vi "rs3_ReadDepthPreference4.vi"(0 "file (use dialog)":path) -> (1 "HDAD 2*":T2={"lambdaCensus"=126.0, "lambdaAD"=800.0, "ignoreSAD"=0}, 2 "ST_AE_Control":cluster{"meanIntensitySetpoint":u32}={"meanIntensitySetpoint"=800}, 3 "ST Color Control 2":T5, 4 "depth control 2":T9={"plusIncrement (47)"=19, "MinusDecrement (46)"=4, "deepSeaMedianThreshold (48)"=554, "scoreThreshA(49)"=1, "scoreThreshB (50)"=632, "textureDifferenceThreshold (52)"=0, "textureCountThreshold (51)"=32, "deepSea2ndPeakThresh.(53)"=665, "deepSeaNeighborThresh.(54)"=126, "IrAgreeThreshold (55)"=11}, 6 "ST RSM 2":T8={"rsmBypass (56)"=0, "diffThresh (57)"=6.49, "sloRauDiffThresh(58)"=0.305, "removeThresh(59)"=60}, 8 "Depth Table":T1={"depthUnits, um"=1000, "depthClampMin"=0, "depthClampMax"=65535, "disparityMultiplier"=0, "disparityShift(0-127)"=0}, 9 "text":string="{\n    \"param-disableraucolor\": 0,\n    \"param-disablesadcolor\": 0,\n    \"param-disablesadnormalize\": 0,\n    \"param-disablesloleftcolor\": 0,\n    \"param-disableslorightcolor\": 0,\n    \"param-lambdaad\": 833,\n    \"param-lambdacensus\": 26,\n    \"param-leftrightthreshold\": 11,\n    \"param-maxscorethreshb\": 632,\n    \"param-medianthreshold\": 554,\n    \"param-minscorethresha\": 1,\n    \"param-neighborthresh\": 126,\n    \"param-raumine\": 7,\n    \"param-rauminn\": 1,\n    \"param-rauminnssum\": 7,\n    \"param-raumins\": 3,\n    \"param-rauminw\": 5,\n    \"param-rauminwesum\": 12,\n    \"param-regioncolorthresholdb\": 0.26379450841061053,\n    \"param-regioncolorthresholdg\": 0.9806201235330119,\n    \"param-regioncolorthresholdr\": 0.013826660558426103,\n    \"param-regionshrinku\": 4,\n    \"param-regionshrinkv\": 1,\n    \"param-regionspatialthresholdu\": 7,\n    \"param-regionspatialthresholdv\": 3,\n    \"param-robbinsmonrodecrement\": 4,\n    \"param-robbinsmonroincrement\": 19,\n    \"param-rsmdiffthreshold\": 1.0367311077984247,\n    \"param-rsmrauslodiffthreshold\": 0.8955340364089305,\n    \"param-rsmremovethreshold\": 0.7604262237190709,\n    \"param-scanlineedgetaub\": 105,\n    \"param-scanlineedgetaug\": 442,\n    \"param-scanlineedgetaur\": 46,\n    \"param-scanlinep1\": 93,\n    \"param-scanlinep1onediscon\": 70,\n    \"param-scanlinep1twodiscon\": 92,\n    \"param-scanlinep2\": 473,\n    \"param-scanlinep2onediscon\": 123,\n    \"param-scanlinep2twodiscon\": 409,\n    \"param-secondpeakdelta\": 665,\n    \"param-texturecountthresh\": 32,\n    \"param-texturedifferencethresh\": 0,\n    \"param-usersm\": 1\n}", 10 "ST SLO Penalty 2":T7={"sloK1Penalty (79)"=10, "sloK2Penalty (80)"=60, "sloK1PenaltyMod1(81)"=84, "sloK2PenaltyMod1(82)"=56, "sloK1PenaltyMod2(83)"=59, "sloK2PenaltyMod2(84)"=4}, 11 "ST_CensusEnable":cluster{"uDiameter":u32, "vDiameter":u32}={"uDiameter"=9, "vDiameter"=9}, 12 "ST SLO Threshold 2":T3={"SLOdiffThreshRed(76)"=200, "SLODiffThreshGreen(77)"=200, "SLODiffThreshBlue(78)"=200}, 13 "error out":errorcluster, 14 "ST Rau Threshold 2":T4={"rauDiffThreshRed(73)"=70, "rauDiffThreshGreen(74)"=70, "rauDiffThreshBlue(75)"=70}, 15 "ST RAU vector 2":T6={"minWest (60)"=7, "minEast (61)"=7, "minWEsum (62)"=12, "minNorth (63)"=3, "minSouth (64)"=2, "minNSSum(65)"=1, "uStrink (66)"=2, "vShrink (67)"=1})   [LabVIEW 2017, in "libRealSense3.lvlib"]
uses:
  libRealSense3.lvlib
panel:
  in  "error in (no error)":errorcluster
  # "RS2 Read Depth Preferences 4"
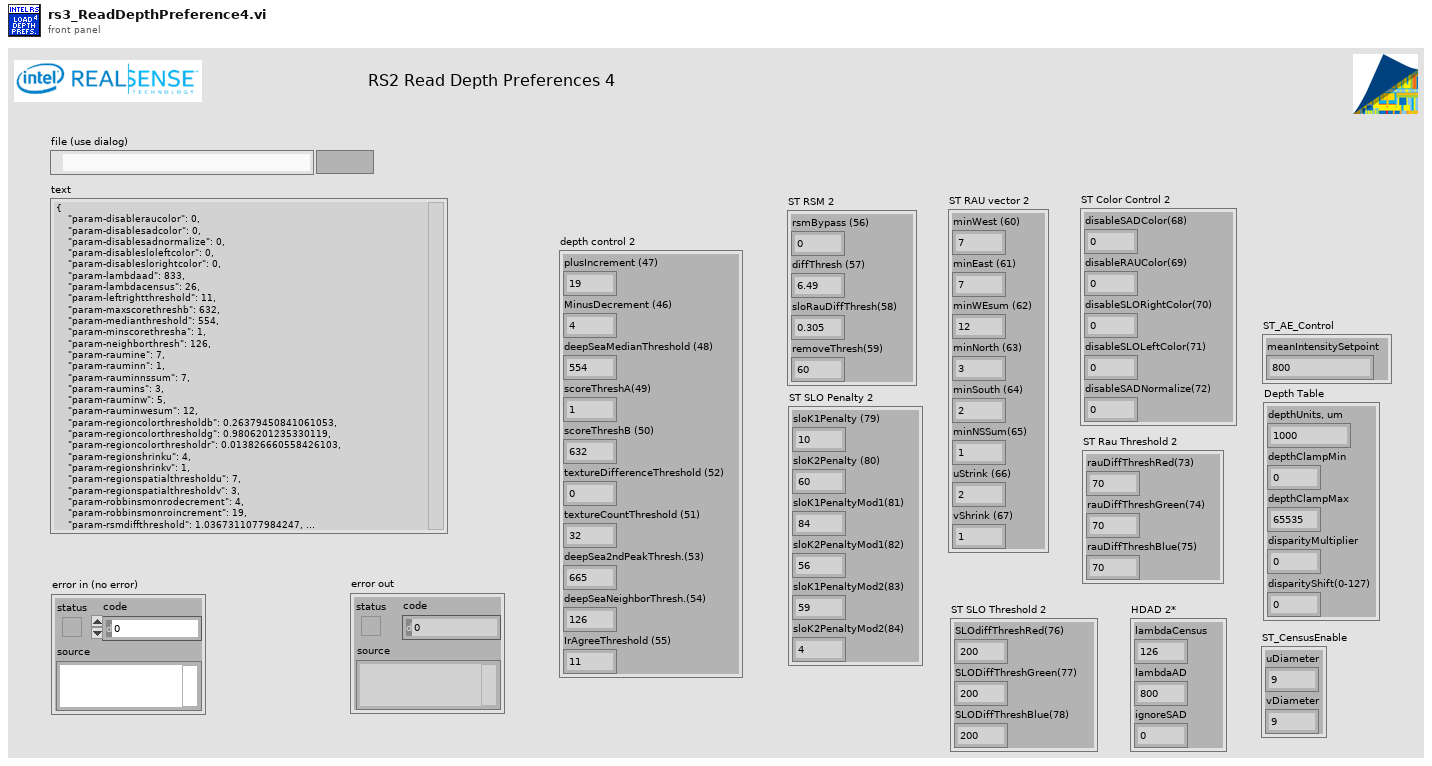
[diagram p1: front panel]
types:
  T1 = cluster{"depthUnits, um":u32, "depthClampMin":u32, "depthClampMax":u32, "disparityMultiplier":u32, "disparityShift(0-127)":u32}
  T2 = cluster{"lambdaCensus":sgl, "lambdaAD":sgl, "ignoreSAD":u32}
  T3 = cluster{"SLOdiffThreshRed(76)":u32, "SLODiffThreshGreen(77)":u32, "SLODiffThreshBlue(78)":u32}
  T4 = cluster{"rauDiffThreshRed(73)":u32, "rauDiffThreshGreen(74)":u32, "rauDiffThreshBlue(75)":u32}
  T5 = cluster{"disableSADColor(68)":u32, "disableRAUColor(69)":u32, "disableSLORightColor(70)":u32, "disableSLOLeftColor(71)":u32, "disableSADNormalize(72)":u32}
  T6 = cluster{"minWest (60)":u32, "minEast (61)":u32, "minWEsum (62)":u32, "minNorth (63)":u32, "minSouth (64)":u32, "minNSSum(65)":u32, "uStrink (66)":u32, "vShrink (67)":u32}
  T7 = cluster{"sloK1Penalty (79)":u32, "sloK2Penalty (80)":u32, "sloK1PenaltyMod1(81)":u32, "sloK2PenaltyMod1(82)":u32, "sloK1PenaltyMod2(83)":u32, "sloK2PenaltyMod2(84)":u32}
  T8 = cluster{"rsmBypass (56)":u32, "diffThresh (57)":sgl, "sloRauDiffThresh(58)":sgl, "removeThresh(59)":u32}
  T9 = cluster{"plusIncrement (47)":u32, "MinusDecrement (46)":u32, "deepSeaMedianThreshold (48)":u32, "scoreThreshA(49)":u32, "scoreThreshB (50)":u32, "textureDifferenceThreshold (52)":u32, "textureCountThreshold (51)":u32, "deepSea2ndPeakThresh.(53)":u32, "deepSeaNeighborThresh.(54)":u32, "IrAgreeThreshold (55)":u32}
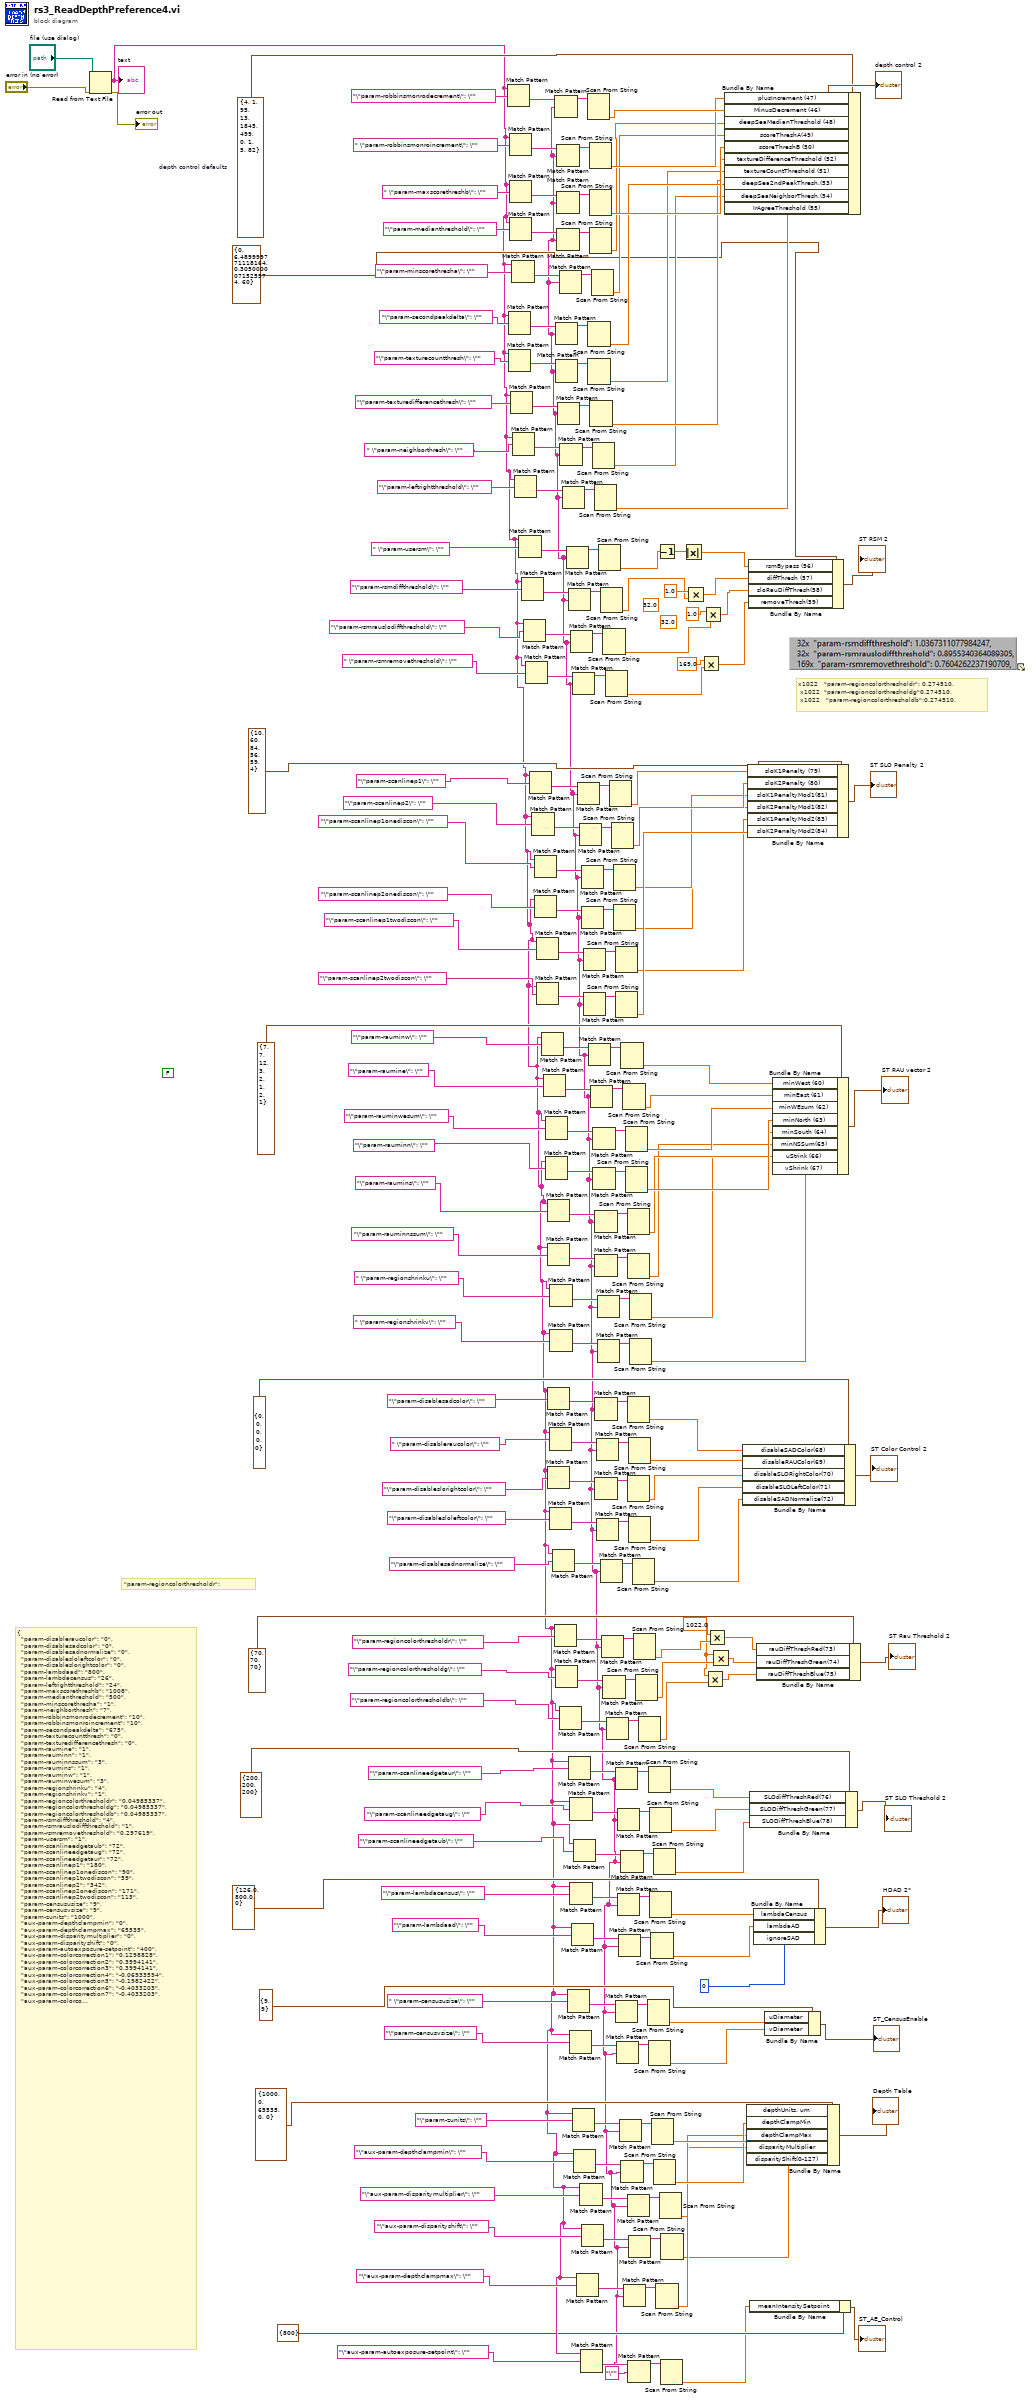
[diagram p0: block diagram]
diagram:
  w1 = "\"" ("regular expression")
  (unwired) 32.0 ("x")
  (unwired) 32.0 ("x")
  w48 = 1022.0
  w229 = T9 {"plusIncrement (47)"=4, "MinusDecrement (46)"=1, "deepSeaMedianThreshold (48)"=95, "scoreThreshA(49)"=13, "scoreThreshB (50)"=1845, "textureDifferenceThreshold (52)"=499, "textureCountThreshold (51)"=0, "deepSea2ndPeakThresh.(53)"=1, "deepSeaNeighborThresh.(54)"=5, "IrAgreeThreshold (55)"=82}  # depth control defaults
  (unwired) FALSE
  # "{\n  \"param-disableraucolor\": \"0\",\n  \"param-disablesadcolor\": \"0\",\n  \"param-disablesadnormalize\": \"0\",\n  \"param-disablesloleftcolor\": \"0\",\n  \"param-disableslorightcolor\": \"0\",\n  \"param-lambdaad\": \"800\",\n  \"param-lambdacensus\": \"26\",\n  \"param-leftrightthreshold\": \"24\",\n  \"param-maxscorethreshb\": \"1008\",\n  \"param-medianthreshold\": \"500\",\n  \"param-minscorethresha\": \"1\",\n  \"param-neighborthresh\": \"7\",\n  \"param-robbinsmonrodecrement\": \"10\",\n  \"param-robbinsmonroincrement\": \"10\",\n  \"param-secondpeakdelta\": \"675\",\n  \"param-texturecountthresh\": \"0\",\n  \"param-texturedifferencethresh\": \"0\",\n  \"param-raumine\": \"1\",\n  \"param-rauminn\": \"1\",\n  \"param-rauminnssum\": \"3\",\n  \"param-raumins\": \"1\",\n  \"param-rauminw\": \"1\",\n  \"param-rauminwesum\": \"3\",\n  \"param-regionshrinku\": \"4\",\n  \"param-regionshrinkv\": \"1\",\n  \"param-regioncolorthresholdr\": \"0.04985337\",\n  \"param-regioncolorthresholdg\": \"0.04985337\",\n  \"param-regioncolorthresholdb\": \"0.04985337\",\n  \"param-rsmdiffthreshold\": \"4\",\n  \"param-rsmrauslodiffthreshold\": \"1\",\n  \"param-rsmremovethreshold\": \"0.297619\",\n  \"param-usersm\": \"1\",\n  \"param-scanlineedgetaub\": \"72\",\n  \"param-scanlineedgetaug\": \"72\",\n  \"param-scanlineedgetaur\": \"72\",\n  \"param-scanlinep1\": \"180\",\n  \"param-scanlinep1onediscon\": \"90\",\n  \"param-scanlinep1twodiscon\": \"59\",\n  \"param-scanlinep2\": \"342\",\n  \"param-scanlinep2onediscon\": \"171\",\n  \"param-scanlinep2twodiscon\": \"113\",\n  \"param-censususize\": \"9\",\n  \"param-censusvsize\": \"9\",\n  \"param-zunits\": \"1000\",\n  \"aux-param-depthclampmin\": \"0\",\n  \"aux-param-depthclampmax\": \"65535\",\n  \"aux-param-disparitymultiplier\": \"0\",\n  \"aux-param-disparityshift\": \"0\",\n  \"aux-param-autoexposure-setpoint\": \"400\",\n  \"aux-param-colorcorrection1\": \"0.1298828\",\n  \"aux-param-colorcorrection2\": \"0.3994141\",\n  \"aux-param-colorcorrection3\": \"0.3994141\",\n  \"aux-param-colorcorrection4\": \"-0.06933594\",\n  \"aux-param-colorcorrection5\": \"-0.1982422\",\n  \"aux-param-colorcorrection6\": \"-0.4033203\",\n  \"aux-param-colorcorrection7\": \"-0.4033203\",\n  \"aux-param-colorcorrection8\": \"1.005859\",\n  \"aux-param-colorcorrection9\": \"0.921875\",\n  \"aux-param-colorcorrection10\": \"-0.4414063\",\n  \"aux-param-colorcorrection11\": \"-0.4414063\",\n  \"aux-param-colorcorrection12\": \"-0.0390625\",\n  \"controls-laserstate\": \"on\",\n  \"controls-laserpower\": \"150\",\n  \"controls-autoexposure-auto\": \"True\",\n  \"controls-autoexposure-manual\": \"33000\"\n}"
  # "x1022   \"param-regioncolorthresholdr\": 0.274510, \n x1022  \"param-regioncolorthresholdg\"0.274510, \n x1022   \"param-regioncolorthresholdb\":0.274510,"
  # "\"param-regioncolorthresholdr\":"
  n1 = Read from Text File(file (use dialog)="file (use dialog)", error in="error in (no error)") -> (text=w5:string, error out=→"error out":errorcluster)  [unwired: 2 in, 2 out]
  "text" <- w5
  n2 = Match Pattern(string=w5, regular expression="\"param-robbinsmonrodecrement\": \"") -> (after substring=w235:string)  [unwired: 1 in, 3 out]
  n3 = Match Pattern(string=w5, regular expression="\"param-secondpeakdelta\": \"") -> (after substring=w210:string)  [unwired: 1 in, 3 out]
  n4 = Match Pattern(string=w5, regular expression="\"param-texturecountthresh\": \"") -> (after substring=w213:string)  [unwired: 1 in, 3 out]
  n5 = Match Pattern(string=w5, regular expression=" \"param-robbinsmonroincrement\": \"") -> (after substring=w232:string)  [unwired: 1 in, 3 out]
  n6 = Match Pattern(string=w5, regular expression=" \"param-maxscorethreshb\": \"") -> (after substring=w225:string)  [unwired: 1 in, 3 out]
  n7 = Match Pattern(string=w5, regular expression="\"param-medianthreshold\": \"") -> (after substring=w222:string)  [unwired: 1 in, 3 out]
  n8 = Match Pattern(string=w5, regular expression="\"param-texturedifferencethresh\": \"") -> (after substring=w214:string)  [unwired: 1 in, 3 out]
  n9 = Match Pattern(string=w5, regular expression="\"param-minscorethresha\": \"") -> (after substring=w221:string)  [unwired: 1 in, 3 out]
  n10 = Match Pattern(string=w5, regular expression=" \"param-neighborthresh\": \"") -> (after substring=w202:string)  [unwired: 1 in, 3 out]
  n11 = Match Pattern(string=w5, regular expression="\"param-leftrightthreshold\": \"") -> (after substring=w201:string)  [unwired: 1 in, 3 out]
  n12 = Match Pattern(string=w5, regular expression=" \"param-usersm\": \"") -> (after substring=w187:string)  [unwired: 1 in, 3 out]
  n13 = Match Pattern(string=w5, regular expression="\"param-rsmdiffthreshold\": \"") -> (after substring=w186:string)  [unwired: 1 in, 3 out]
  n14 = Match Pattern(string=w5, regular expression="\"param-rsmrauslodiffthreshold\": \"") -> (after substring=w190:string)  [unwired: 1 in, 3 out]
  n15 = Match Pattern(string=w5, regular expression=" \"param-rsmremovethreshold\": \"") -> (after substring=w191:string)  [unwired: 1 in, 3 out]
  n16 = Match Pattern(string=w5, regular expression="\"param-scanlinep1\": \"") -> (after substring=w176:string)  [unwired: 1 in, 3 out]
  n17 = Match Pattern(string=w5, regular expression="\"param-scanlinep2\": \"") -> (after substring=w174:string)  [unwired: 1 in, 3 out]
  n18 = Match Pattern(string=w5, regular expression="\"param-scanlinep1onediscon\": \"") -> (after substring=w173:string)  [unwired: 1 in, 3 out]
  n19 = Match Pattern(string=w5, regular expression="\"param-scanlinep2onediscon\": \"") -> (after substring=w170:string)  [unwired: 1 in, 3 out]
  n20 = Match Pattern(string=w5, regular expression="\"param-scanlinep1twodiscon\": \"") -> (after substring=w169:string)  [unwired: 1 in, 3 out]
  n21 = Match Pattern(string=w5, regular expression="\"param-scanlinep2twodiscon\": \"") -> (after substring=w162:string)  [unwired: 1 in, 3 out]
  n22 = Match Pattern(string=w5, regular expression="\"param-rauminw\": \"") -> (after substring=w139:string)  [unwired: 1 in, 3 out]
  n23 = Match Pattern(string=w5, regular expression="\"param-raumine\": \"") -> (after substring=w141:string)  [unwired: 1 in, 3 out]
  n24 = Match Pattern(string=w5, regular expression="\"param-rauminwesum\": \"") -> (after substring=w142:string)  [unwired: 1 in, 3 out]
  n25 = Match Pattern(string=w5, regular expression="\"param-rauminn\": \"") -> (after substring=w145:string)  [unwired: 1 in, 3 out]
  n26 = Match Pattern(string=w5, regular expression="\"param-raumins\": \"") -> (after substring=w146:string)  [unwired: 1 in, 3 out]
  n27 = Match Pattern(string=w5, regular expression="\"param-rauminnssum\": \"") -> (after substring=w149:string)  [unwired: 1 in, 3 out]
  n28 = Match Pattern(string=w5, regular expression="\"param-disablesadcolor\": \"") -> (after substring=w115:string)  [unwired: 1 in, 3 out]
  n29 = Match Pattern(string=w5, regular expression="\"param-disableslorightcolor\": \"") -> (after substring=w108:string)  [unwired: 1 in, 3 out]
  n30 = Match Pattern(string=w5, regular expression=" \"param-disableraucolor\": \"") -> (after substring=w112:string)  [unwired: 1 in, 3 out]
  n31 = Match Pattern(string=w5, regular expression="\"param-disablesloleftcolor\": \"") -> (after substring=w111:string)  [unwired: 1 in, 3 out]
  n32 = Match Pattern(string=w5, regular expression=" \"param-regionshrinku\": \"") -> (after substring=w137:string)  [unwired: 1 in, 3 out]
  n33 = Match Pattern(string=w5, regular expression=" \"param-regionshrinkv\": \"") -> (after substring=w134:string)  [unwired: 1 in, 3 out]
  n34 = Match Pattern(string=w5, regular expression="\"param-disablesadnormalize\": \"") -> (after substring=w106:string)  [unwired: 1 in, 3 out]
  n35 = Match Pattern(string=w5, regular expression="\"param-regioncolorthresholdr\": \"") -> (after substring=w92:string)  [unwired: 1 in, 3 out]
  n36 = Match Pattern(string=w235, regular expression=w1) -> (before substring=w236:string)  [unwired: 1 in, 3 out]
  n37 = Match Pattern(string=w210, regular expression=w1) -> (before substring=w211:string)  [unwired: 1 in, 3 out]
  n38 = Match Pattern(string=w213, regular expression=w1) -> (before substring=w212:string)  [unwired: 1 in, 3 out]
  n39 = Match Pattern(string=w5, regular expression="\"param-regioncolorthresholdg\": \"") -> (after substring=w89:string)  [unwired: 1 in, 3 out]
  n40 = Match Pattern(string=w232, regular expression=w1) -> (before substring=w231:string)  [unwired: 1 in, 3 out]
  n41 = Match Pattern(string=w225, regular expression=w1) -> (before substring=w224:string)  [unwired: 1 in, 3 out]
  n42 = Match Pattern(string=w222, regular expression=w1) -> (before substring=w223:string)  [unwired: 1 in, 3 out]
  n43 = Match Pattern(string=w214, regular expression=w1) -> (before substring=w215:string)  [unwired: 1 in, 3 out]
  n44 = Match Pattern(string=w221, regular expression=w1) -> (before substring=w220:string)  [unwired: 1 in, 3 out]
  n45 = Match Pattern(string=w5, regular expression="\"param-regioncolorthresholdb\": \"") -> (after substring=w94:string)  [unwired: 1 in, 3 out]
  n46 = Match Pattern(string=w202, regular expression=w1) -> (before substring=w203:string)  [unwired: 1 in, 3 out]
  n47 = Match Pattern(string=w201, regular expression=w1) -> (before substring=w200:string)  [unwired: 1 in, 3 out]
  n48 = Match Pattern(string=w187, regular expression=w1) -> (before substring=w188:string)  [unwired: 1 in, 3 out]
  n49 = Match Pattern(string=w5, regular expression=" \"param-censususize\": \"") -> (after substring=w35:string)  [unwired: 1 in, 3 out]
  n50 = Match Pattern(string=w186, regular expression=w1) -> (before substring=w185:string)  [unwired: 1 in, 3 out]
  n51 = Match Pattern(string=w5, regular expression="\"param-scanlineedgetaur\": \"") -> (after substring=w82:string)  [unwired: 1 in, 3 out]
  n52 = Match Pattern(string=w5, regular expression="\"param-censusvsize\": \"") -> (after substring=w38:string)  [unwired: 1 in, 3 out]
  n53 = Match Pattern(string=w5, regular expression="\"param-scanlineedgetaug\": \"") -> (after substring=w85:string)  [unwired: 1 in, 3 out]
  n54 = Match Pattern(string=w5, regular expression="\"param-lambdacensus\": \"") -> (after substring=w76:string)  [unwired: 1 in, 3 out]
  n55 = Match Pattern(string=w190, regular expression=w1) -> (before substring=w189:string)  [unwired: 1 in, 3 out]
  n56 = Match Pattern(string=w5, regular expression="\"param-lambdaad\": \"") -> (after substring=w73:string)  [unwired: 1 in, 3 out]
  n57 = Match Pattern(string=w5, regular expression="\"param-zunits\": \"") -> (after substring=w28:string)  [unwired: 1 in, 3 out]
  n58 = Match Pattern(string=w191, regular expression=w1) -> (before substring=w192:string)  [unwired: 1 in, 3 out]
  n59 = Match Pattern(string=w5, regular expression="\"param-scanlineedgetaub\": \"") -> (after substring=w80:string)  [unwired: 1 in, 3 out]
  n60 = Match Pattern(string=w5, regular expression="\"aux-param-depthclampmin\": \"") -> (after substring=w25:string)  [unwired: 1 in, 3 out]
  n61 = Match Pattern(string=w5, regular expression="\"aux-param-depthclampmax\": \"") -> (after substring=w15:string)  [unwired: 1 in, 3 out]
  n62 = Match Pattern(string=w176, regular expression=w1) -> (before substring=w177:string)  [unwired: 1 in, 3 out]
  n63 = Match Pattern(string=w174, regular expression=w1) -> (before substring=w175:string)  [unwired: 1 in, 3 out]
  n64 = Match Pattern(string=w5, regular expression="\"aux-param-disparitymultiplier\": \"") -> (after substring=w17:string)  [unwired: 1 in, 3 out]
  n65 = Match Pattern(string=w5, regular expression="\"aux-param-autoexposure-setpoint\": \"") -> (after substring=w7:string)  [unwired: 1 in, 3 out]
  n66 = Match Pattern(string=w173, regular expression=w1) -> (before substring=w172:string)  [unwired: 1 in, 3 out]
  n67 = Match Pattern(string=w170, regular expression=w1) -> (before substring=w171:string)  [unwired: 1 in, 3 out]
  n68 = Match Pattern(string=w5, regular expression="\"aux-param-disparityshift\": \"") -> (after substring=w20:string)  [unwired: 1 in, 3 out]
  n69 = Match Pattern(string=w169, regular expression=w1) -> (before substring=w168:string)  [unwired: 1 in, 3 out]
  n70 = Match Pattern(string=w162, regular expression=w1) -> (before substring=w163:string)  [unwired: 1 in, 3 out]
  n71 = Scan From String(input string=w236) -> (output 1=w228:dbl)  [unwired: 4 in, 3 out]
  n72 = Scan From String(input string=w211) -> (output 1=w206:dbl)  [unwired: 4 in, 3 out]
  n73 = Scan From String(input string=w212) -> (output 1=w205:dbl)  [unwired: 4 in, 3 out]
  n74 = Match Pattern(string=w139, regular expression=w1) -> (before substring=w138:string)  [unwired: 1 in, 3 out]
  n75 = Scan From String(input string=w231) -> (output 1=w227:dbl)  [unwired: 4 in, 3 out]
  n76 = Scan From String(input string=w224) -> (output 1=w218:dbl)  [unwired: 4 in, 3 out]
  n77 = Scan From String(input string=w223) -> (output 1=w216:dbl)  [unwired: 4 in, 3 out]
  n78 = Scan From String(input string=w215) -> (output 1=w204:dbl)  [unwired: 4 in, 3 out]
  n79 = Match Pattern(string=w141, regular expression=w1) -> (before substring=w140:string)  [unwired: 1 in, 3 out]
  n80 = Scan From String(input string=w220) -> (output 1=w217:dbl)  [unwired: 4 in, 3 out]
  n81 = Scan From String(input string=w203) -> (output 1=w198:dbl)  [unwired: 4 in, 3 out]
  n82 = Match Pattern(string=w142, regular expression=w1) -> (before substring=w143:string)  [unwired: 1 in, 3 out]
  n83 = Match Pattern(string=w145, regular expression=w1) -> (before substring=w144:string)  [unwired: 1 in, 3 out]
  n84 = Scan From String(input string=w200) -> (output 1=w195:dbl)  [unwired: 4 in, 3 out]
  n85 = Match Pattern(string=w146, regular expression=w1) -> (before substring=w147:string)  [unwired: 1 in, 3 out]
  n86 = Match Pattern(string=w149, regular expression=w1) -> (before substring=w148:string)  [unwired: 1 in, 3 out]
  n87 = Match Pattern(string=w115, regular expression=w1) -> (before substring=w114:string)  [unwired: 1 in, 3 out]
  n88 = Match Pattern(string=w108, regular expression=w1) -> (before substring=w109:string)  [unwired: 1 in, 3 out]
  n89 = Match Pattern(string=w112, regular expression=w1) -> (before substring=w113:string)  [unwired: 1 in, 3 out]
  n90 = Match Pattern(string=w111, regular expression=w1) -> (before substring=w110:string)  [unwired: 1 in, 3 out]
  n91 = Match Pattern(string=w137, regular expression=w1) -> (before substring=w136:string)  [unwired: 1 in, 3 out]
  n92 = Match Pattern(string=w134, regular expression=w1) -> (before substring=w135:string)  [unwired: 1 in, 3 out]
  n93 = Scan From String(input string=w188) -> (output 1=w178:dbl)  [unwired: 4 in, 3 out]
  n94 = Match Pattern(string=w106, regular expression=w1) -> (before substring=w107:string)  [unwired: 1 in, 3 out]
  n95 = Scan From String(input string=w185) -> (output 1=w46:dbl)  [unwired: 4 in, 3 out]
  n96 = Match Pattern(string=w92, regular expression=w1) -> (before substring=w91:string)  [unwired: 1 in, 3 out]
  n97 = Scan From String(input string=w189) -> (output 1=w65:dbl)  [unwired: 4 in, 3 out]
  n98 = Match Pattern(string=w89, regular expression=w1) -> (before substring=w90:string)  [unwired: 1 in, 3 out]
  n99 = Scan From String(input string=w192) -> (output 1=w43:dbl)  [unwired: 4 in, 3 out]
  n100 = Match Pattern(string=w94, regular expression=w1) -> (before substring=w93:string)  [unwired: 1 in, 3 out]
  n101 = Scan From String(input string=w177) -> (output 1=w159:dbl)  [unwired: 4 in, 3 out]
  n102 = Scan From String(input string=w175) -> (output 1=w158:dbl)  [unwired: 4 in, 3 out]
  n103 = Scan From String(input string=w172) -> (output 1=w157:dbl)  [unwired: 4 in, 3 out]
  n104 = Scan From String(input string=w171) -> (output 1=w153:dbl)  [unwired: 4 in, 3 out]
  n105 = Match Pattern(string=w35, regular expression=w1) -> (before substring=w36:string)  [unwired: 1 in, 3 out]
  n106 = Scan From String(input string=w168) -> (output 1=w152:dbl)  [unwired: 4 in, 3 out]
  n107 = Scan From String(input string=w163) -> (output 1=w160:dbl)  [unwired: 4 in, 3 out]
  n108 = Match Pattern(string=w82, regular expression=w1) -> (before substring=w83:string)  [unwired: 1 in, 3 out]
  n109 = Match Pattern(string=w38, regular expression=w1) -> (before substring=w37:string)  [unwired: 1 in, 3 out]
  n110 = Match Pattern(string=w85, regular expression=w1) -> (before substring=w84:string)  [unwired: 1 in, 3 out]
  n111 = Match Pattern(string=w76, regular expression=w1) -> (before substring=w75:string)  [unwired: 1 in, 3 out]
  n112 = Match Pattern(string=w73, regular expression=w1) -> (before substring=w74:string)  [unwired: 1 in, 3 out]
  n113 = Match Pattern(string=w28, regular expression=w1) -> (before substring=w27:string)  [unwired: 1 in, 3 out]
  n114 = Scan From String(input string=w138) -> (output 1=w133:dbl)  [unwired: 4 in, 3 out]
  n115 = Match Pattern(string=w80, regular expression=w1) -> (before substring=w81:string)  [unwired: 1 in, 3 out]
  n116 = Match Pattern(string=w25, regular expression=w1) -> (before substring=w26:string)  [unwired: 1 in, 3 out]
  n117 = Scan From String(input string=w140) -> (output 1=w132:dbl)  [unwired: 4 in, 3 out]
  n118 = Match Pattern(string=w15, regular expression=w1) -> (before substring=w16:string)  [unwired: 1 in, 3 out]
  n119 = Scan From String(input string=w143) -> (output 1=w131:dbl)  [unwired: 4 in, 3 out]
  n120 = Scan From String(input string=w144) -> (output 1=w130:dbl)  [unwired: 4 in, 3 out]
  n121 = Scan From String(input string=w147) -> (output 1=w129:dbl)  [unwired: 4 in, 3 out]
  n122 = Scan From String(input string=w148) -> (output 1=w128:dbl)  [unwired: 4 in, 3 out]
  n123 = Scan From String(input string=w114) -> (output 1=w105:dbl)  [unwired: 4 in, 3 out]
  n124 = Scan From String(input string=w109) -> (output 1=w103:dbl)  [unwired: 4 in, 3 out]
  n125 = Match Pattern(string=w17, regular expression=w1) -> (before substring=w18:string)  [unwired: 1 in, 3 out]
  n126 = Match Pattern(string=w7, regular expression=w1) -> (before substring=w6:string)  [unwired: 1 in, 3 out]
  n127 = Scan From String(input string=w113) -> (output 1=w104:dbl)  [unwired: 4 in, 3 out]
  n128 = Scan From String(input string=w110) -> (output 1=w102:dbl)  [unwired: 4 in, 3 out]
  n129 = Match Pattern(string=w20, regular expression=w1) -> (before substring=w19:string)  [unwired: 1 in, 3 out]
  n130 = Scan From String(input string=w136) -> (output 1=w127:dbl)  [unwired: 4 in, 3 out]
  n131 = Scan From String(input string=w135) -> (output 1=w126:dbl)  [unwired: 4 in, 3 out]
  n132 = Scan From String(input string=w107) -> (output 1=w101:dbl)  [unwired: 4 in, 3 out]
  n133 = Scan From String(input string=w91) -> (output 1=w54:dbl)  [unwired: 4 in, 3 out]
  n134 = Scan From String(input string=w90) -> (output 1=w52:dbl)  [unwired: 4 in, 3 out]
  n135 = Scan From String(input string=w93) -> (output 1=w49:dbl)  [unwired: 4 in, 3 out]
  n136 = Scan From String(input string=w36) -> (output 1=w33:dbl)  [unwired: 4 in, 3 out]
  n137 = Scan From String(input string=w83) -> (output 1=w79:dbl)  [unwired: 4 in, 3 out]
  n138 = Scan From String(input string=w37) -> (output 1=w32:dbl)  [unwired: 4 in, 3 out]
  n139 = Scan From String(input string=w84) -> (output 1=w78:dbl)  [unwired: 4 in, 3 out]
  n140 = Scan From String(input string=w75) -> (output 1=w68:dbl)  [unwired: 4 in, 3 out]
  n141 = Scan From String(input string=w74) -> (output 1=w67:dbl)  [unwired: 4 in, 3 out]
  n142 = Scan From String(input string=w27) -> (output 1=w13:dbl)  [unwired: 4 in, 3 out]
  n143 = Scan From String(input string=w81) -> (output 1=w77:dbl)  [unwired: 4 in, 3 out]
  n144 = Scan From String(input string=w26) -> (output 1=w12:dbl)  [unwired: 4 in, 3 out]
  n145 = Decrement(x=w178) -> (x-1=w179:dbl)
  n146 = Scan From String(input string=w16) -> (output 1=w11:dbl)  [unwired: 4 in, 3 out]
  n147 = Scan From String(input string=w18) -> (output 1=w10:dbl)  [unwired: 4 in, 3 out]
  n148 = Scan From String(input string=w6) -> (output 1=w2:dbl)  [unwired: 4 in, 3 out]
  n149 = Scan From String(input string=w19) -> (output 1=w9:dbl)  [unwired: 4 in, 3 out]
  n150 = Absolute Value(x=w179) -> (abs(x)=w180:dbl)
  n151 = Multiply(x=1.0, y=w46) -> (x*y=w45:dbl)
  n152 = Multiply(x=169.0, y=w43) -> (x*y=w42:dbl)
  n153 = Multiply(x=1.0, y=w65) -> (x*y=w63:dbl)
  n154 = Multiply(x=w48, y=w49) -> (x*y=w50:dbl)
  n155 = Multiply(x=w48, y=w54) -> (x*y=w53:dbl)
  n156 = Multiply(x=w48, y=w52) -> (x*y=w51:dbl)
  n157 = Bundle By Name(cluster=w229, "plusIncrement (47)"=w227, "MinusDecrement (46)"=w228, "deepSeaMedianThreshold (48)"=w216, "scoreThreshA(49)"=w217, "scoreThreshB (50)"=w218, "textureDifferenceThreshold (52)"=w204, "textureCountThreshold (51)"=w205, "deepSea2ndPeakThresh.(53)"=w206, "deepSeaNeighborThresh.(54)"=w198, "IrAgreeThreshold (55)"=w195) -> (→"depth control 2":T9)
  n158 = Bundle By Name(cluster=T5 {"disableSADColor(68)"=0, "disableRAUColor(69)"=0, "disableSLORightColor(70)"=0, "disableSLOLeftColor(71)"=0, "disableSADNormalize(72)"=0} ("ST Color Control 2"), "disableSADColor(68)"=w105, "disableRAUColor(69)"=w104, "disableSLORightColor(70)"=w103, "disableSLOLeftColor(71)"=w102, "disableSADNormalize(72)"=w101) -> (→"ST Color Control 2":T5)
  n159 = Bundle By Name(cluster=T1 {"depthUnits, um"=1000, "depthClampMin"=0, "depthClampMax"=65535, "disparityMultiplier"=0, "disparityShift(0-127)"=0} ("Depth Table"), "depthUnits, um"=w13, "depthClampMin"=w12, "depthClampMax"=w11, "disparityMultiplier"=w10, "disparityShift(0-127)"=w9) -> (→"Depth Table":T1)
  n160 = Bundle By Name(cluster=T7 {"sloK1Penalty (79)"=10, "sloK2Penalty (80)"=60, "sloK1PenaltyMod1(81)"=84, "sloK2PenaltyMod1(82)"=56, "sloK1PenaltyMod2(83)"=59, "sloK2PenaltyMod2(84)"=4} ("ST SLO Penalty 2"), "sloK1Penalty (79)"=w159, "sloK2Penalty (80)"=w158, "sloK1PenaltyMod1(81)"=w157, "sloK2PenaltyMod1(82)"=w153, "sloK1PenaltyMod2(83)"=w152, "sloK2PenaltyMod2(84)"=w160) -> (→"ST SLO Penalty 2":T7)
  n161 = Bundle By Name(cluster=T8 {"rsmBypass (56)"=0, "diffThresh (57)"=6.49, "sloRauDiffThresh(58)"=0.305, "removeThresh(59)"=60} ("ST RSM 2"), "rsmBypass (56)"=w180, "diffThresh (57)"=w45, "sloRauDiffThresh(58)"=w63, "removeThresh(59)"=w42) -> (→"ST RSM 2":T8)
  n162 = Bundle By Name(cluster=cluster{"meanIntensitySetpoint":u32} {"meanIntensitySetpoint"=800} ("ST_AE_Control"), "meanIntensitySetpoint"=w2) -> (→"ST_AE_Control":cluster{"meanIntensitySetpoint":u32})
  n163 = Bundle By Name(cluster=T3 {"SLOdiffThreshRed(76)"=200, "SLODiffThreshGreen(77)"=200, "SLODiffThreshBlue(78)"=200} ("ST SLO Threshold 2"), "SLOdiffThreshRed(76)"=w79, "SLODiffThreshGreen(77)"=w78, "SLODiffThreshBlue(78)"=w77) -> (→"ST SLO Threshold 2":T3)
  n164 = Bundle By Name(cluster=T2 {"lambdaCensus"=126.0, "lambdaAD"=800.0, "ignoreSAD"=0} ("HDAD 2*"), "lambdaCensus"=w68, "lambdaAD"=w67, "ignoreSAD"=u32 0) -> (→"HDAD 2*":T2)
  n165 = Bundle By Name(cluster=T4 {"rauDiffThreshRed(73)"=70, "rauDiffThreshGreen(74)"=70, "rauDiffThreshBlue(75)"=70} ("ST Rau Threshold 2"), "rauDiffThreshRed(73)"=w53, "rauDiffThreshGreen(74)"=w51, "rauDiffThreshBlue(75)"=w50) -> (→"ST Rau Threshold 2":T4)
  n166 = Bundle By Name(cluster=cluster{"uDiameter":u32, "vDiameter":u32} {"uDiameter"=9, "vDiameter"=9} ("ST_CensusEnable"), "uDiameter"=w33, "vDiameter"=w32) -> (→"ST_CensusEnable":cluster{"uDiameter":u32, "vDiameter":u32})
  n167 = Bundle By Name(cluster=T6 {"minWest (60)"=7, "minEast (61)"=7, "minWEsum (62)"=12, "minNorth (63)"=3, "minSouth (64)"=2, "minNSSum(65)"=1, "uStrink (66)"=2, "vShrink (67)"=1} ("ST RAU vector 2"), "minWest (60)"=w133, "minEast (61)"=w132, "minWEsum (62)"=w131, "minNorth (63)"=w130, "minSouth (64)"=w129, "minNSSum(65)"=w128, "uStrink (66)"=w127, "vShrink (67)"=w126) -> (→"ST RAU vector 2":T6)
